vi "App - analyze RUS V6.vi"() -> ()   [LabVIEW 2018] (continued)
"z(inf)"=-0.13064639987627175-0.4414329201397408i, "z (pi/2)"=0.4734329201397408-0.15464639987627177i, "z center"=0.028000000000000025+0.0040000000000000036i, "z(0)"=0.1866463998762718+0.4494329201397408i, "radius"=0.4728415871493524}}, "timestamp(min)"=474.80000000447035, "timestamp"=timestamp(3493756309 s since 1904-01-01), "Magn Field(T)"=0.0}, {"temperature"=120.365, "lorentzian"={"A (VHz)"=0.00010643307998407587, "f (Hz)"=668.3129997886653, "G (Hz)"=0.026481266968947207, "phi(rad)"=2.884384764495416, "Q"=25237.19883086979, "Norm  Ampl"=0.01202799865082056, "bg (V)"=-0.12754197010931823-0.42726620706178137i, "4corners"={"z (-pi/2)"=-0.4512662070617814+0.12754197010931823i, "z(inf)"=-0.12754197010931823-0.42726620706178137i, "z (pi/2)"=0.42726620706178137-0.10354197010931819i, "z center"=-0.01200000000000001+0.01200000000000001i, "z(0)"=0.10354197010931819+0.4512662070617814i, "radius"=0.4542078241545233}}, "timestamp(min)"=476.1166666671634, "timestamp"=timestamp(3493756388 s since 1904-01-01), "Magn Field(T)"=0.0}, {"temperature"=120.108, "lorentzian"={"A (VHz)"=9.976743757357866e-05, "f (Hz)"=668.3140680165973, "G (Hz)"=0.02490702053107623, "phi(rad)"=3.037932161061489, "Q"=26832.35705301438, "Norm  Ampl"=0.011771320920466868, "bg (V)"=-0.020903351691279173-0.4660736150774217i, "4corners"={"z (-pi/2)"=-0.44207361507742166+0.0529033516912792i, "z(inf)"=-0.020903351691279173-0.4660736150774217i, "z (pi/2)"=0.4980736150774217-0.044903351691279195i, "z center"=0.028000000000000025+0.0040000000000000036i, "z(0)"=0.07690335169127922+0.4740736150774217i, "radius"=0.4726105599736393}}, "timestamp(min)"=477.45000000298023, "timestamp"=timestamp(3493756468 s since 1904-01-01), "Magn Field(T)"=0.0}, {"temperature"=119.859, "lorentzian"={"A (VHz)"=0.00011898875098084783, "f (Hz)"=668.3088794677242, "G (Hz)"=0.029414461497605328, "phi(rad)"=3.1937111533621003, "Q"=22720.418645846436, "Norm  Ampl"=0.014251449395847925, "bg (V)"=0.0612402357051023-0.4798469642263822i, "4corners"={"z (-pi/2)"=-0.44784696422638215-0.02124023570510226i, "z(inf)"=0.0612402357051023-0.4798469642263822i, "z (pi/2)"=0.5198469642263822+0.029240235705102268i, "z center"=0.03600000000000003+0.0040000000000000036i, "z(0)"=0.010759764294897767+0.4878469642263822i, "radius"=0.4845048547636392}}, "timestamp(min)"=478.76666666567326, "timestamp"=timestamp(3493756547 s since 1904-01-01), "Magn Field(T)"=0.0}, {"temperature"=119.604, "lorentzian"={"A (VHz)"=0.00010355482355173766, "f (Hz)"=668.3109415026871, "G (Hz)"=0.02529392336725071, "phi(rad)"=3.2924075486690434, "Q"=26421.798303065247, "Norm  Ampl"=0.011934347555654482, "bg (V)"=0.10688904433211106-0.4624709498016203i, "4corners"={"z (-pi/2)"=-0.43047094980162026-0.06688904433211103i, "z(inf)"=0.10688904433211106-0.4624709498016203i, "z (pi/2)"=0.5024709498016203+0.07488904433211103i, "z center"=0.03600000000000003+0.0040000000000000036i, "z(0)"=-0.034889044332111+0.4704709498016203i, "radius"=0.4718266669182082}}, "timestamp(min)"=480.08333333581686, "timestamp"=timestamp(3493756626 s since 1904-01-01), "Magn Field(T)"=0.0}, {"temperature"=119.349, "lorentzian"={"A (VHz)"=8.801887306847703e-05, "f (Hz)"=668.3052156629583, "G (Hz)"=0.021698735780586516, "phi(rad)"=3.2142167974714875, "Q"=30799.26970956895, "Norm  Ampl"=0.010466488120373691, "bg (V)"=0.07099981492336191-0.47708326828925746i, "4corners"={"z (-pi/2)"=-0.4450832682892574-0.03099981492336188i, "z(inf)"=0.07099981492336191-0.47708326828925746i, "z (pi/2)"=0.5170832682892574+0.03899981492336189i, "z center"=0.03600000000000003+0.0040000000000000036i, "z(0)"=0.0010001850766381479+0.48508326828925746i, "radius"=0.48235474297714054}}, "timestamp(min)"=481.41666666418314, "timestamp"=timestamp(3493756706 s since 1904-01-01), "Magn Field(T)"=0.0}, {"temperature"=119.104, "lorentzian"={"A (VHz)"=0.00010821801624048861, "f (Hz)"=668.3064621156966, "G (Hz)"=0.025882538370321603, "phi(rad)"=3.375797533755535, "Q"=25820.74650305609, "Norm  Ampl"=0.012706744245672173, "bg (V)"=0.14993201098301023-0.4735358362984421i, "4corners"={"z (-pi/2)"=-0.44153583629844206-0.1099320109830102i, "z(inf)"=0.14993201098301023-0.4735358362984421i, "z (pi/2)"=0.5135358362984421+0.1179320109830102i, "z center"=0.03600000000000003+0.0040000000000000036i, "z(0)"=-0.07793201098301017+0.4815358362984421i, "radius"=0.49093887407281694}}, "timestamp(min)"=482.73333333432674, "timestamp"=timestamp(3493756785 s since 1904-01-01), "Magn Field(T)"=0.0}, {"temperature"=118.85, "lorentzian"={"A (VHz)"=9.39701073854705e-05, "f (Hz)"=668.2991530946135, "G (Hz)"=0.022918275642981233, "phi(rad)"=3.2389285611028322, "Q"=29160.09753549157, "Norm  Ampl"=0.011143619731764974, "bg (V)"=0.08325322342802156-0.4799313693938589i, "4corners"={"z (-pi/2)"=-0.44793136939385886-0.04325322342802153i, "z(inf)"=0.08325322342802156-0.4799313693938589i, "z (pi/2)"=0.519931369393859+0.051253223428021535i, "z center"=0.03600000000000003+0.0040000000000000036i, "z(0)"=-0.0112532234280215+0.4879313693938589i, "radius"=0.48623290448894346}}, "timestamp(min)"=484.0666666701436, "timestamp"=timestamp(3493756865 s since 1904-01-01), "Magn Field(T)"=0.0}, {"temperature"=118.609, "lorentzian"={"A (VHz)"=0.00010743883910296562, "f (Hz)"=668.296337187602, "G (Hz)"=0.026266437532917148, "phi(rad)"=3.235613845829878, "Q"=25442.975902236147, "Norm  Ampl"=0.012711224583429891, "bg (V)"=0.08143305323019587-0.4777966817581062i, "4corners"={"z (-pi/2)"=-0.44579668175810616-0.041433053230195825i, "z(inf)"=0.08143305323019587-0.4777966817581062i, "z (pi/2)"=0.5177966817581062+0.04943305323019583i, "z center"=0.03600000000000003+0.0040000000000000036i, "z(0)"=-0.009433053230195797+0.4857966817581062i, "radius"=0.4839340914617813}}, "timestamp(min)"=485.3833333328366, "timestamp"=timestamp(3493756944 s since 1904-01-01), "Magn Field(T)"=0.0}, {"temperature"=118.359, "lorentzian"={"A (VHz)"=0.0001070844718829983, "f (Hz)"=668.2941712628873, "G (Hz)"=0.026124370760870142, "phi(rad)"=3.33110736221513, "Q"=25581.25427709356, "Norm  Ampl"=0.012647127694562135, "bg (V)"=0.13519818462181604-0.4714445853921451i, "4corners"={"z (-pi/2)"=-0.4314445853921451-0.08719818462181601i, "z(inf)"=0.13519818462181604-0.4714445853921451i, "z (pi/2)"=0.5194445853921452+0.09519818462181602i, "z center"=0.04400000000000004+0.0040000000000000036i, "z(0)"=-0.04719818462181598+0.47944458539214513i, "radius"=0.48411224179628387}}, "timestamp(min)"=486.70000000298023, "timestamp"=timestamp(3493757023 s since 1904-01-01), "Magn Field(T)"=0.0}, {"temperature"=118.111, "lorentzian"={"A (VHz)"=0.0001130613397389126, "f (Hz)"=668.2879323748828, "G (Hz)"=0.02790011297894843, "phi(rad)"=3.2373022589244065, "Q"=23952.875491189887, "Norm  Ampl"=0.013424939419339223, "bg (V)"=0.08198314261289943-0.47497648031024303i, "4corners"={"z (-pi/2)"=-0.442976480310243-0.04198314261289939i, "z(inf)"=0.08198314261289943-0.47497648031024303i, "z (pi/2)"=0.514976480310243+0.0499831426128994i, "z center"=0.03600000000000003+0.0040000000000000036i, "z(0)"=-0.009983142612899364+0.48297648031024304i, "radius"=0.4811786758522731}}, "timestamp(min)"=488.0333333313465, "timestamp"=timestamp(3493757103 s since 1904-01-01), "Magn Field(T)"=0.0}, {"temperature"=117.87, "lorentzian"={"A (VHz)"=0.00011059651751790313, "f (Hz)"=668.2827006729923, "G (Hz)"=0.027979379247465956, "phi(rad)"=3.139826857303401, "Q"=23884.82942249398, "Norm  Ampl"=0.013390188683237079, "bg (V)"=0.03515493717875207-0.4745727263376128i, "4corners"={"z (-pi/2)"=-0.4425727263376128+0.004845062821247961i, "z(inf)"=0.03515493717875207-0.4745727263376128i, "z (pi/2)"=0.5145727263376129+0.0031549371787520457i, "z center"=0.03600000000000003+0.0040000000000000036i, "z(0)"=0.03684506282124799+0.48257272633761283i, "radius"=0.47857347244220244}}, "timestamp(min)"=489.3500000014901, "timestamp"=timestamp(3493757182 s since 1904-01-01), "Magn Field(T)"=0.0}, {"temperature"=117.621, "lorentzian"={"A (VHz)"=0.00011421298073050124, "f (Hz)"=668.2752935986506, "G (Hz)"=0.02906321623228526, "phi(rad)"=3.0733097507748752, "Q"=22993.85203129336, "Norm  Ampl"=0.01393302684205042, "bg (V)"=0.003290324428110697-0.4742869727474171i, "4corners"={"z (-pi/2)"=-0.4422869727474171+0.03670967557188934i, "z(inf)"=0.003290324428110697-0.4742869727474171i, "z (pi/2)"=0.5142869727474171-0.02870967557188933i, "z center"=0.03600000000000003+0.0040000000000000036i, "z(0)"=0.06870967557188937+0.4822869727474171i, "radius"=0.4794041626601784}}, "timestamp(min)"=490.66666666418314, "timestamp"=timestamp(3493757261 s since 1904-01-01), "Magn Field(T)"=0.0}, {"temperature"=117.382, "lorentzian"={"A (VHz)"=0.00011070346840073388, "f (Hz)"=668.2706731525243, "G (Hz)"=0.028260232808520972, "phi(rad)"=3.0887902740086197, "Q"=23647.033542874018, "Norm  Ampl"=0.013444461231823078, "bg (V)"=0.010891582862682068-0.47107476262981013i, "4corners"={"z (-pi/2)"=-0.4390747626298101+0.029108417137317967i, "z(inf)"=0.010891582862682068-0.47107476262981013i, "z (pi/2)"=0.5110747626298102-0.02110841713731796i, "z center"=0.03600000000000003+0.0040000000000000036i, "z(0)"=0.061108417137317995+0.47907476262981014i, "radius"=0.4757378087759181}}, "timestamp(min)"=492.0, "timestamp"=timestamp(3493757341 s since 1904-01-01), "Magn Field(T)"=0.0}, {"temperature"=117.138, "lorentzian"={"A (VHz)"=0.00010800943974293567, "f (Hz)"=668.265311084802, "G (Hz)"=0.02797683885251187, "phi(rad)"=3.0873037764057782, "Q"=23886.37667778547, "Norm  Ampl"=0.013306749021252626, "bg (V)"=0.010191020561799904-0.4709337312500312i, "4corners"={"z (-pi/2)"=-0.43893373125003116+0.029808979438200132i, "z(inf)"=0.010191020561799904-0.4709337312500312i, "z (pi/2)"=0.5109337312500313-0.021808979438200125i, "z center"=0.03600000000000003+0.0040000000000000036i, "z(0)"=0.06180897943820016+0.4789337312500312i, "radius"=0.4756344736230946}}, "timestamp(min)"=493.3166666701436, "timestamp"=timestamp(3493757420 s since 1904-01-01), "Magn Field(T)"=0.0}, {"temperature"=116.892, "lorentzian"={"A (VHz)"=0.00011678085083385915, "f (Hz)"=668.2583083453824, "G (Hz)"=0.03012977871709603, "phi(rad)"=3.0862999154696142, "Q"=22179.330111249834, "Norm  Ampl"=0.014575891093322855, "bg (V)"=0.00926464512112294-0.47903094309897204i, "4corners"={"z (-pi/2)"=-0.447030943098972+0.030735354878877096i, "z(inf)"=0.00926464512112294-0.47903094309897204i, "z (pi/2)"=0.5190309430989721-0.02273535487887709i, "z center"=0.03600000000000003+0.0040000000000000036i, "z(0)"=0.06273535487887713+0.48703094309897205i, "radius"=0.48377026695693265}}, "timestamp(min)"=494.6499999985099, "timestamp"=timestamp(3493757500 s since 1904-01-01), "Magn Field(T)"=0.0}, {"temperature"=116.657, "lorentzian"={"A (VHz)"=0.00012538810354815837, "f (Hz)"=668.2568309954227, "G (Hz)"=0.032286617496826396, "phi(rad)"=3.2130369520804023, "Q"=20697.64140084073, "Norm  Ampl"=0.015358626788303374, "bg (V)"=0.06195688871592034-0.4704828421346862i, "4corners"={"z (-pi/2)"=-0.4464828421346862-0.02995688871592031i, "z(inf)"=0.06195688871592034-0.4704828421346862i, "z (pi/2)"=0.5024828421346863+0.03795688871592032i, "z center"=0.028000000000000025+0.0040000000000000036i, "z(0)"=-0.005956888715920289+0.4784828421346862i, "radius"=0.4756963714087748}}, "timestamp(min)"=495.9666666686535, "timestamp"=timestamp(3493757579 s since 1904-01-01), "Magn Field(T)"=0.0}, {"temperature"=116.414, "lorentzian"={"A (VHz)"=0.00012730750637721753, "f (Hz)"=668.251544958297, "G (Hz)"=0.03283669747483084, "phi(rad)"=3.262105480773335, "Q"=20350.753770853735, "Norm  Ampl"=0.015732228210800864, "bg (V)"=0.09359864898441411-0.47163017441834365i, "4corners"={"z (-pi/2)"=-0.4396301744183436-0.05359864898441408i, "z(inf)"=0.09359864898441411-0.47163017441834365i, "z (pi/2)"=0.5116301744183437+0.061598648984414084i, "z center"=0.03600000000000003+0.0040000000000000036i, "z(0)"=-0.02159864898441405+0.47963017441834366i, "radius"=0.47910506904232786}}, "timestamp(min)"=497.2833333313465, "timestamp"=timestamp(3493757658 s since 1904-01-01), "Magn Field(T)"=0.0}, {"temperature"=116.182, "lorentzian"={"A (VHz)"=0.00013443649190837575, "f (Hz)"=668.2453085062731, "G (Hz)"=0.035201673002130396, "phi(rad)"=3.27100569161246, "Q"=18983.33946985506, "Norm  Ampl"=0.016690935833129323, "bg (V)"=0.0971902879419883-0.4661868320027308i, "4corners"={"z (-pi/2)"=-0.4341868320027308-0.05719028794198826i, "z(inf)"=0.0971902879419883-0.4661868320027308i, "z (pi/2)"=0.5061868320027308+0.06519028794198826i, "z center"=0.03600000000000003+0.0040000000000000036i, "z(0)"=-0.02519028794198823+0.4741868320027308i, "radius"=0.4741517777328138}}, "timestamp(min)"=498.6166666671634, "timestamp"=timestamp(3493757738 s since 1904-01-01), "Magn Field(T)"=0.0}, {"temperature"=115.94, "lorentzian"={"A (VHz)"=0.0001411771983919197, "f (Hz)"=668.2394743021457, "G (Hz)"=0.0369135267967175, "phi(rad)"=3.2980610919863382, "Q"=18102.83471373882, "Norm  Ampl"=0.017546101039359215, "bg (V)"=0.11007101432524297-0.46552310715567025i, "4corners"={"z (-pi/2)"=-0.4335231071556702-0.07007101432524293i, "z(inf)"=0.11007101432524297-0.46552310715567025i, "z (pi/2)"=0.5055231071556703+0.07807101432524294i, "z center"=0.03600000000000003+0.0040000000000000036i, "z(0)"=-0.0380710143252429+0.47352310715567025i, "radius"=0.4753298468603516}}, "timestamp(min)"=499.933333337307, "timestamp"=timestamp(3493757817 s since 1904-01-01), "Magn Field(T)"=0.0}, {"temperature"=115.7, "lorentzian"={"A (VHz)"=0.0001435934643755886, "f (Hz)"=668.2322266809226, "G (Hz)"=0.03813748540583941, "phi(rad)"=3.3056536907773015, "Q"=17521.664566238192, "Norm  Ampl"=0.01822797887630577, "bg (V)"=0.114062403211538-0.4675364967002526i, "4corners"={"z (-pi/2)"=-0.4355364967002526-0.07406240321153797i, "z(inf)"=0.114062403211538-0.4675364967002526i, "z (pi/2)"=0.5075364967002527+0.08206240321153797i, "z center"=0.03600000000000003+0.0040000000000000036i, "z(0)"=-0.04206240321153794+0.4755364967002526i, "radius"=0.47795439794556555}}, "timestamp(min)"=501.25, "timestamp"=timestamp(3493757896 s since 1904-01-01), "Magn Field(T)"=0.0}, {"temperature"=115.472, "lorentzian"={"A (VHz)"=0.00015015013294900263, "f (Hz)"=668.2226032955875, "G (Hz)"=0.03977315572948954, "phi(rad)"=3.294194856757234, "Q"=16800.84446505557, "Norm  Ampl"=0.019165843957809636, "bg (V)"=0.1092507018179084-0.47227890465981215i, "4corners"={"z (-pi/2)"=-0.4402789046598121-0.06925070181790836i, "z(inf)"=0.1092507018179084-0.47227890465981215i, "z (pi/2)"=0.5122789046598122+0.07725070181790837i, "z center"=0.03600000000000003+0.0040000000000000036i, "z(0)"=-0.037250701817908335+0.48027890465981216i, "radius"=0.4818788855519264}}, "timestamp(min)"=502.58333333581686, "timestamp"=timestamp(3493757976 s since 1904-01-01), "Magn Field(T)"=0.0}, {"temperature"=115.231, "lorentzian"={"A (VHz)"=0.000152798278466846, "f (Hz)"=668.2221912502285, "G (Hz)"=0.040622965881621786, "phi(rad)"=3.3489762299985824, "Q"=16449.369876081317, "Norm  Ampl"=0.019466830319116384, "bg (V)"=0.1346689441843829-0.46493952367230446i, "4corners"={"z (-pi/2)"=-0.4329395236723044-0.09466894418438287i, "z(inf)"=0.1346689441843829-0.46493952367230446i, "z (pi/2)"=0.5049395236723044+0.10266894418438288i, "z center"=0.03600000000000003+0.0040000000000000036i, "z(0)"=-0.06266894418438285+0.47293952367230446i, "radius"=0.4792075097580052}}, "timestamp(min)"=503.8999999985099, "timestamp"=timestamp(3493758055 s since 1904-01-01), "Magn Field(T)"=0.0}, {"temperature"=115.003, "lorentzian"={"A (VHz)"=0.00015016084801885404, "f (Hz)"=668.2178106776172, "G (Hz)"=0.039990622388638174, "phi(rad)"=3.381149177122383, "Q"=16709.36261465803, "Norm  Ampl"=0.019131967464758187, "bg (V)"=0.15751353904588636-0.4607494937776951i, "4corners"={"z (-pi/2)"=-0.42074949377769505-0.10951353904588632i, "z(inf)"=0.15751353904588636-0.4607494937776951i, "z (pi/2)"=0.5087494937776951+0.11751353904588632i, "z center"=0.04400000000000004+0.0040000000000000036i, "z(0)"=-0.06951353904588628+0.4687494937776951i, "radius"=0.47841134551068687}}, "timestamp(min)"=505.23333333432674, "timestamp"=timestamp(3493758135 s since 1904-01-01), "Magn Field(T)"=0.0}, {"temperature"=114.767, "lorentzian"={"A (VHz)"=0.00015757298754621695, "f (Hz)"=668.2137975862624, "G (Hz)"=0.04267438204697135, "phi(rad)"=3.4106089120816963, "Q"=15658.429379264706, "Norm  Ampl"=0.02049382198056047, "bg (V)"=0.16363895936930345-0.458964339411539i, "4corners"={"z (-pi/2)"=-0.426964339411539-0.12363895936930341i, "z(inf)"=0.16363895936930345-0.458964339411539i, "z (pi/2)"=0.49896433941153906+0.13163895936930342i, "z center"=0.03600000000000003+0.0040000000000000036i, "z(0)"=-0.09163895936930339+0.46696433941153903i, "radius"=0.4802371117642215}}, "timestamp(min)"=506.55000000447035, "timestamp"=timestamp(3493758214 s since 1904-01-01), "Magn Field(T)"=0.0}, {"temperature"=114.531, "lorentzian"={"A (VHz)"=0.00015361317354396095, "f (Hz)"=668.2079346540519, "G (Hz)"=0.041298080432760224, "phi(rad)"=3.398310296093033, "Q"=16180.120907604885, "Norm  Ampl"=0.01996843308490766, "bg (V)"=0.16676908728823442-0.463674027337198i, "4corners"={"z (-pi/2)"=-0.42367402733719794-0.11876908728823439i, "z(inf)"=0.16676908728823442-0.463674027337198i, "z (pi/2)"=0.511674027337198+0.12676908728823438i, "z center"=0.04400000000000004+0.0040000000000000036i, "z(0)"=-0.07876908728823435+0.471674027337198i, "radius"=0.48351964245455464}}, "timestamp(min)"=507.8666666671634, "timestamp"=timestamp(3493758293 s since 1904-01-01), "Magn Field(T)"=0.0}, {"temperature"=114.307, "lorentzian"={"A (VHz)"=0.00015578562086982487, "f (Hz)"=668.2000760755379, "G (Hz)"=0.04298628045116837, "phi(rad)"=3.383233224979629, "Q"=15544.496268631594, "Norm  Ampl"=0.02045395031435505, "bg (V)"=0.14186296929284245-0.45800079061954285i, "4corners"={"z (-pi/2)"=-0.43400079061954283-0.10986296929284242i, "z(inf)"=0.14186296929284245-0.45800079061954285i, "z (pi/2)"=0.4900007906195429+0.11786296929284243i, "z center"=0.028000000000000025+0.0040000000000000036i, "z(0)"=-0.0858629692928424+0.46600079061954286i, "radius"=0.475825079529511}}, "timestamp(min)"=509.20000000298023, "timestamp"=timestamp(3493758373 s since 1904-01-01), "Magn Field(T)"=0.0}, {"temperature"=114.072, "lorentzian"={"A (VHz)"=0.00015529053749936577, "f (Hz)"=668.194062828963, "G (Hz)"=0.041694845458546674, "phi(rad)"=3.3543260153288053, "Q"=16025.819390391709, "Norm  Ampl"=0.01973127159447459, "bg (V)"=0.14391430053991824-0.458562662430859i, "4corners"={"z (-pi/2)"=-0.418562662430859-0.0959143005399182i, "z(inf)"=0.14391430053991824-0.458562662430859i, "z (pi/2)"=0.506562662430859+0.10391430053991821i, "z center"=0.04400000000000004+0.0040000000000000036i, "z(0)"=-0.055914300539918166+0.46656266243085903i, "radius"=0.47323047675261354}}, "timestamp(min)"=510.51666666567326, "timestamp"=timestamp(3493758452 s since 1904-01-01), "Magn Field(T)"=0.0}, {"temperature"=113.842, "lorentzian"={"A (VHz)"=0.00016067612699950575, "f (Hz)"=668.1891261636409, "G (Hz)"=0.042796849003211866, "phi(rad)"=3.394809062342997, "Q"=15613.044925655482, "Norm  Ampl"=0.020075211030941627, "bg (V)"=0.15351387700829827-0.45012328964369214i, "4corners"={"z (-pi/2)"=-0.4181232896436921-0.11351387700829825i, "z(inf)"=0.15351387700829827-0.45012328964369214i, "z (pi/2)"=0.4901232896436922+0.12151387700829826i, "z center"=0.03600000000000003+0.0040000000000000036i, "z(0)"=-0.08151387700829822+0.45812328964369214i, "radius"=0.46908152115205964}}, "timestamp(min)"=511.8500000014901, "timestamp"=timestamp(3493758532 s since 1904-01-01), "Magn Field(T)"=0.0}, {"temperature"=113.618, "lorentzian"={"A (VHz)"=0.0001542811582452129, "f (Hz)"=668.1800061469135, "G (Hz)"=0.040982167537354335, "phi(rad)"=3.3443220525752206, "Q"=16304.164623256744, "Norm  Ampl"=0.01923169205406682, "bg (V)"=0.1384844541906579-0.45565943755480826i, "4corners"={"z (-pi/2)"=-0.4156594375548082-0.09048445419065788i, "z(inf)"=0.1384844541906579-0.45565943755480826i, "z (pi/2)"=0.5036594375548082+0.09848445419065789i, "z center"=0.04400000000000004+0.0040000000000000036i, "z(0)"=-0.05048445419065785+0.46365943755480826i, "radius"=0.4692697631607104}}, "timestamp(min)"=513.1666666641831, "timestamp"=timestamp(3493758611 s since 1904-01-01), "Magn Field(T)"=0.0}, {"temperature"=113.387, "lorentzian"={"A (VHz)"=0.0001624912168982803, "f (Hz)"=668.1744243080439, "G (Hz)"=0.044416582325911676, "phi(rad)"=3.3737772248575197, "Q"=15043.355191204013, "Norm  Ampl"=0.020891572072933687, "bg (V)"=0.1442306313832896-0.4537337421361339i, "4corners"={"z (-pi/2)"=-0.42173374213613385-0.10423063138328956i, "z(inf)"=0.1442306313832896-0.4537337421361339i, "z (pi/2)"=0.4937337421361339+0.11223063138328956i, "z center"=0.03600000000000003+0.0040000000000000036i, "z(0)"=-0.07223063138328953+0.4617337421361339i, "radius"=0.47035523624126285}}, "timestamp(min)"=514.4833333343267, "timestamp"=timestamp(3493758690 s since 1904-01-01), "Magn Field(T)"=0.0}, {"temperature"=113.167, "lorentzian"={"A (VHz)"=0.0001556983032149633, "f (Hz)"=668.167621356464, "G (Hz)"=0.042992225411489386, "phi(rad)"=3.348175213684548, "Q"=15541.591879956524, "Norm  Ampl"=0.020129996156841454, "bg (V)"=0.1240404082002707-0.45426853495999503i, "4corners"={"z (-pi/2)"=-0.430268534959995-0.09204040820027067i, "z(inf)"=0.1240404082002707-0.45426853495999503i, "z (pi/2)"=0.48626853495999506+0.10004040820027067i, "z center"=0.028000000000000025+0.0040000000000000036i, "z(0)"=-0.06804040820027064+0.46226853495999504i, "radius"=0.4682241024783483}}, "timestamp(min)"=515.8000000044703, "timestamp"=timestamp(3493758769 s since 1904-01-01), "Magn Field(T)"=0.0}, {"temperature"=112.937, "lorentzian"={"A (VHz)"=0.00016419580746214888, "f (Hz)"=668.1637736220466, "G (Hz)"=0.045224329465811286, "phi(rad)"=3.425485977825887, "Q"=14774.431849280716, "Norm  Ampl"=0.0213288848716954, "bg (V)"=0.1680996752259816-0.44874605720083394i, "4corners"={"z (-pi/2)"=-0.4167460572008339-0.12809967522598156i, "z(inf)"=0.1680996752259816-0.44874605720083394i, "z (pi/2)"=0.48874605720083397+0.13609967522598157i, "z center"=0.03600000000000003+0.0040000000000000036i, "z(0)"=-0.09609967522598153+0.45674605720083394i, "radius"=0.4716241262973202}}, "timestamp(min)"=517.1333333328366, "timestamp"=timestamp(3493758849 s since 1904-01-01), "Magn Field(T)"=0.0}, {"temperature"=112.71, "lorentzian"={"A (VHz)"=0.00017245504712525025, "f (Hz)"=668.1572968562582, "G (Hz)"=0.047433759727580925, "phi(rad)"=3.4412811422325076, "Q"=14086.112943472835, "Norm  Ampl"=0.02252752294707743, "bg (V)"=0.1762088681702268-0.4497577792019217i, "4corners"={"z (-pi/2)"=-0.4177577792019217-0.13620886817022676i, "z(inf)"=0.1762088681702268-0.4497577792019217i, "z (pi/2)"=0.48975777920192176+0.14420886817022677i, "z center"=0.03600000000000003+0.0040000000000000036i, "z(0)"=-0.10420886817022673+0.45775777920192173i, "radius"=0.4749259404368601}}, "timestamp(min)"=518.4500000029802, "timestamp"=timestamp(3493758928 s since 1904-01-01), "Magn Field(T)"=0.0}, {"temperature"=112.492, "lorentzian"={"A (VHz)"=0.00017070211204150683, "f (Hz)"=668.1537550879266, "G (Hz)"=0.04677378805996331, "phi(rad)"=3.473672889865301, "Q"=14284.79032383187, "Norm  Ampl"=0.022093838974345924, "bg (V)"=0.18999264751515837-0.44254858424220067i, "4corners"={"z (-pi/2)"=-0.41054858424220064-0.14999264751515834i, "z(inf)"=0.18999264751515837-0.44254858424220067i, "z (pi/2)"=0.4825485842422007+0.15799264751515835i, "z center"=0.03600000000000003+0.0040000000000000036i, "z(0)"=-0.11799264751515831+0.4505485842422007i, "radius"=0.4723551350175434}}, "timestamp(min)"=519.7666666656733, "timestamp"=timestamp(3493759007 s since 1904-01-01), "Magn Field(T)"=0.0}, {"temperature"=112.266, "lorentzian"={"A (VHz)"=0.00018223977875365084, "f (Hz)"=668.1449838049871, "G (Hz)"=0.049945994320608485, "phi(rad)"=3.5026596091685995, "Q"=13377.348732234572, "Norm  Ampl"=0.02355087112785759, "bg (V)"=0.20257746875969504-0.4451228845478489i, "4corners"={"z (-pi/2)"=-0.40512288454784884-0.170577468759695i, "z(inf)"=0.20257746875969504-0.4451228845478489i, "z (pi/2)"=0.4771228845478489+0.162577468759695i, "z center"=0.03600000000000003-0.0040000000000000036i, "z(0)"=-0.13057746875969498+0.43712288454784887i, "radius"=0.4715267249798276}}, "timestamp(min)"=521.1000000014901, "timestamp"=timestamp(3493759087 s since 1904-01-01), "Magn Field(T)"=0.0}, {"temperature"=112.049, "lorentzian"={"A (VHz)"=0.00017118504286424681, "f (Hz)"=668.135169475204, "G (Hz)"=0.04711813776736462, "phi(rad)"=3.4409139299761327, "Q"=14179.999489240714, "Norm  Ampl"=0.021846821113515342, "bg (V)"=0.18072038464819612-0.4390447280498502i, "4corners"={"z (-pi/2)"=-0.39904472804985014-0.13272038464819608i, "z(inf)"=0.18072038464819612-0.4390447280498502i, "z (pi/2)"=0.4870447280498502+0.14072038464819608i, "z center"=0.04400000000000004+0.0040000000000000036i, "z(0)"=-0.09272038464819604+0.4470447280498502i, "radius"=0.46366053814306474}}, "timestamp(min)"=522.4166666641831, "timestamp"=timestamp(3493759166 s since 1904-01-01), "Magn Field(T)"=0.0}, {"temperature"=111.826, "lorentzian"={"A (VHz)"=0.0001799658759591542, "f (Hz)"=668.1246913482574, "G (Hz)"=0.049217323444046425, "phi(rad)"=3.414889237193867, "Q"=13574.99036102251, "Norm  Ampl"=0.02301194999389016, "bg (V)"=0.17019722104335014-0.44620515508772524i, "4corners"={"z (-pi/2)"=-0.4062051550877252-0.1221972210433501i, "z(inf)"=0.17019722104335014-0.44620515508772524i, "z (pi/2)"=0.4942051550877253+0.1301972210433501i, "z center"=0.04400000000000004+0.0040000000000000036i, "z(0)"=-0.08219722104335006+0.45420515508772524i, "radius"=0.4675579325245449}}, "timestamp(min)"=523.7333333343267, "timestamp"=timestamp(3493759245 s since 1904-01-01), "Magn Field(T)"=0.0}, {"temperature"=111.603, "lorentzian"={"A (VHz)"=0.00017451974083226369, "f (Hz)"=668.121193286822, "G (Hz)"=0.047920841140946836, "phi(rad)"=3.4354084610725897, "Q"=13942.184180818429, "Norm  Ampl"=0.022112608133803717, "bg (V)"=0.16963616531755749-0.4376656445815023i, "4corners"={"z (-pi/2)"=-0.4056656445815023-0.12963616531755745i, "z(inf)"=0.16963616531755749-0.4376656445815023i, "z (pi/2)"=0.47766564458150235+0.13763616531755746i, "z center"=0.03600000000000003+0.0040000000000000036i, "z(0)"=-0.09763616531755742+0.4456656445815023i, "radius"=0.46144031714228817}}, "timestamp(min)"=525.0666666701436, "timestamp"=timestamp(3493759325 s since 1904-01-01), "Magn Field(T)"=0.0}, {"temperature"=111.388, "lorentzian"={"A (VHz)"=0.00018136247232028246, "f (Hz)"=668.1101664128744, "G (Hz)"=0.05012247702670941, "phi(rad)"=3.4571429929100543, "Q"=13329.55205020793, "Norm  Ampl"=0.02324003286140558, "bg (V)"=0.17989361626749142-0.4447717760991525i, "4corners"={"z (-pi/2)"=-0.4047717760991525-0.1478936162674914i, "z(inf)"=0.17989361626749142-0.4447717760991525i, "z (pi/2)"=0.47677177609915256+0.1398936162674914i, "z center"=0.03600000000000003-0.0040000000000000036i, "z(0)"=-0.10789361626749136+0.4367717760991525i, "radius"=0.4636648912826348}}, "timestamp(min)"=526.3833333328366, "timestamp"=timestamp(3493759404 s since 1904-01-01), "Magn Field(T)"=0.0}, {"temperature"=111.168, "lorentzian"={"A (VHz)"=0.00017732924367748604, "f (Hz)"=668.0998885496297, "G (Hz)"=0.04886431968750325, "phi(rad)"=3.424337305450411, "Q"=13672.550704118205, "Norm  Ampl"=0.02270721472310118, "bg (V)"=0.17364755516380617-0.44224762483338026i, "4corners"={"z (-pi/2)"=-0.4022476248333802-0.12564755516380613i, "z(inf)"=0.17364755516380617-0.44224762483338026i, "z (pi/2)"=0.4902476248333803+0.13364755516380614i, "z center"=0.04400000000000004+0.0040000000000000036i, "z(0)"=-0.0856475551638061+0.45024762483338027i, "radius"=0.46469929118666137}}, "timestamp(min)"=527.7166666686535, "timestamp"=timestamp(3493759484 s since 1904-01-01), "Magn Field(T)"=0.0}, {"temperature"=110.956, "lorentzian"={"A (VHz)"=0.0001755500351100679, "f (Hz)"=668.0911411970284, "G (Hz)"=0.04871683645184766, "phi(rad)"=3.448905477042299, "Q"=13713.762835511254, "Norm  Ampl"=0.022606833604015622, "bg (V)"=0.1763730746007246-0.43830500659198746i, "4corners"={"z (-pi/2)"=-0.4063050065919874-0.13637307460072456i, "z(inf)"=0.1763730746007246-0.43830500659198746i, "z (pi/2)"=0.4783050065919875+0.14437307460072457i, "z center"=0.03600000000000003+0.0040000000000000036i, "z(0)"=-0.10437307460072454+0.44630500659198746i, "radius"=0.46404560005370016}}, "timestamp(min)"=529.0333333313465, "timestamp"=timestamp(3493759563 s since 1904-01-01), "Magn Field(T)"=0.0}, {"temperature"=110.737, "lorentzian"={"A (VHz)"=0.00018163078790725488, "f (Hz)"=668.0843412935199, "G (Hz)"=0.05044469627537442, "phi(rad)"=3.4720539578691874, "Q"=13243.896596115665, "Norm  Ampl"=0.023423640340629357, "bg (V)"=0.18666973329833123-0.4352186583969567i, "4corners"={"z (-pi/2)"=-0.4032186583969567-0.1466697332983312i, "z(inf)"=0.18666973329833123-0.4352186583969567i, "z (pi/2)"=0.47521865839695676+0.1546697332983312i, "z center"=0.03600000000000003+0.0040000000000000036i, "z(0)"=-0.11466973329833116+0.44321865839695673i, "radius"=0.46434297498316135}}, "timestamp(min)"=530.3500000014901, "timestamp"=timestamp(3493759642 s since 1904-01-01), "Magn Field(T)"=0.0}, {"temperature"=110.519, "lorentzian"={"A (VHz)"=0.0001812071541479742, "f (Hz)"=668.074848351984, "G (Hz)"=0.04959100517706317, "phi(rad)"=3.468032582893634, "Q"=13471.694029323324, "Norm  Ampl"=0.02311847271252755, "bg (V)"=0.1934922330292432-0.4375636507764309i, "4corners"={"z (-pi/2)"=-0.39756365077643085-0.14549223302924316i, "z(inf)"=0.1934922330292432-0.4375636507764309i, "z (pi/2)"=0.48556365077643093+0.15349223302924317i, "z center"=0.04400000000000004+0.0040000000000000036i, "z(0)"=-0.10549223302924313+0.4455636507764309i, "radius"=0.46618278113104883}}, "timestamp(min)"=531.683333337307, "timestamp"=timestamp(3493759722 s since 1904-01-01), "Magn Field(T)"=0.0}, {"temperature"=110.309, "lorentzian"={"A (VHz)"=0.00018694349041188402, "f (Hz)"=668.0672099835513, "G (Hz)"=0.051848808398743444, "phi(rad)"=3.473847235715632, "Q"=12884.909617319998, "Norm  Ampl"=0.02422816607882838, "bg (V)"=0.1964167197133136-0.43772880401937153i, "4corners"={"z (-pi/2)"=-0.3977288040193715-0.14841671971331355i, "z(inf)"=0.1964167197133136-0.43772880401937153i, "z (pi/2)"=0.4857288040193716+0.15641671971331356i, "z center"=0.04400000000000004+0.0040000000000000036i, "z(0)"=-0.10841671971331351+0.44572880401937154i, "radius"=0.4672849160293441}}, "timestamp(min)"=533.0, "timestamp"=timestamp(3493759801 s since 1904-01-01), "Magn Field(T)"=0.0}, {"temperature"=110.092, "lorentzian"={"A (VHz)"=0.0001795295724214495, "f (Hz)"=668.0546726344026, "G (Hz)"=0.04925847870413864, "phi(rad)"=3.448860296676748, "Q"=13562.22705631941, "Norm  Ampl"=0.022840883312951803, "bg (V)"=0.17624688448219566-0.4379766471865395i, "4corners"={"z (-pi/2)"=-0.4059766471865395-0.13624688448219563i, "z(inf)"=0.17624688448219566-0.4379766471865395i, "z (pi/2)"=0.47797664718653954+0.14424688448219564i, "z center"=0.03600000000000003+0.0040000000000000036i, "z(0)"=-0.1042468844821956+0.4459766471865395i, "radius"=0.4636944524848417}}, "timestamp(min)"=534.3166666701436, "timestamp"=timestamp(3493759880 s since 1904-01-01), "Magn Field(T)"=0.0}, {"temperature"=109.886, "lorentzian"={"A (VHz)"=0.00018425700947939067, "f (Hz)"=668.0432151630731, "G (Hz)"=0.05082571027386269, "phi(rad)"=3.474109311678734, "Q"=13143.804809878216, "Norm  Ampl"=0.02335282091786171, "bg (V)"=0.18598107581107173-0.43030073113085054i, "4corners"={"z (-pi/2)"=-0.3983007311308505-0.1459810758110717i, "z(inf)"=0.18598107581107173-0.43030073113085054i, "z (pi/2)"=0.4703007311308506+0.1539810758110717i, "z center"=0.03600000000000003+0.0040000000000000036i, "z(0)"=-0.11398107581107167+0.43830073113085055i, "radius"=0.45946865852007557}}, "timestamp(min)"=535.6499999985099, "timestamp"=timestamp(3493759960 s since 1904-01-01), "Magn Field(T)"=0.0}, {"temperature"=109.672, "lorentzian"={"A (VHz)"=0.00017864747951855305, "f (Hz)"=668.0317886551247, "G (Hz)"=0.04953081680635286, "phi(rad)"=3.4551378676700635, "Q"=13487.195078306127, "Norm  Ampl"=0.022852422995206817, "bg (V)"=0.17830413376772314-0.4348838990750027i, "4corners"={"z (-pi/2)"=-0.40288389907500266-0.1383041337677231i, "z(inf)"=0.17830413376772314-0.4348838990750027i, "z (pi/2)"=0.4748838990750027+0.1463041337677231i, "z center"=0.03600000000000003+0.0040000000000000036i, "z(0)"=-0.10630413376772307+0.4428838990750027i, "radius"=0.4613778747996692}}, "timestamp(min)"=536.9666666686535, "timestamp"=timestamp(3493760039 s since 1904-01-01), "Magn Field(T)"=0.0}, {"temperature"=109.459, "lorentzian"={"A (VHz)"=0.00018219936447157122, "f (Hz)"=668.0206931728633, "G (Hz)"=0.05023590564749462, "phi(rad)"=3.441928253257153, "Q"=13297.673935857052, "Norm  Ampl"=0.023329381688540478, "bg (V)"=0.17338744962959346-0.43960889542050224i, "4corners"={"z (-pi/2)"=-0.4076088954205022-0.13338744962959342i, "z(inf)"=0.17338744962959346-0.43960889542050224i, "z (pi/2)"=0.4796088954205023+0.14138744962959343i, "z center"=0.03600000000000003+0.0040000000000000036i, "z(0)"=-0.1013874496295934+0.44760889542050225i, "radius"=0.46439655835494964}}, "timestamp(min)"=538.3000000044703, "timestamp"=timestamp(3493760119 s since 1904-01-01), "Magn Field(T)"=0.0}, {"temperature"=109.253, "lorentzian"={"A (VHz)"=0.00018326309436219655, "f (Hz)"=668.0108019958866, "G (Hz)"=0.05071614794503111, "phi(rad)"=3.4752117285047524, "Q"=13171.560322757805, "Norm  Ampl"=0.023314289131758165, "bg (V)"=0.1865360113880276-0.43835512614416294i, "4corners"={"z (-pi/2)"=-0.3983551261441629-0.15453601138802758i, "z(inf)"=0.1865360113880276-0.43835512614416294i, "z (pi/2)"=0.47035512614416297+0.14653601138802758i, "z center"=0.03600000000000003-0.0040000000000000036i, "z(0)"=-0.11453601138802755+0.43035512614416294i, "radius"=0.45970149698726026}}, "timestamp(min)"=539.6166666671634, "timestamp"=timestamp(3493760198 s since 1904-01-01), "Magn Field(T)"=0.0}, {"temperature"=109.04, "lorentzian"={"A (VHz)"=0.00017757199001747914, "f (Hz)"=668.000884305955, "G (Hz)"=0.049458648389355514, "phi(rad)"=3.4510272008382445, "Q"=13506.250293118039, "Norm  Ampl"=0.022916329744467515, "bg (V)"=0.17709732027014569-0.4373371638070479i, "4corners"={"z (-pi/2)"=-0.4053371638070479-0.13709732027014565i, "z(inf)"=0.17709732027014569-0.4373371638070479i, "z (pi/2)"=0.47733716380704794+0.14509732027014566i, "z center"=0.03600000000000003+0.0040000000000000036i, "z(0)"=-0.10509732027014562+0.4453371638070479i, "radius"=0.46334322693297797}}, "timestamp(min)"=540.933333337307, "timestamp"=timestamp(3493760277 s since 1904-01-01), "Magn Field(T)"=0.0}, {"temperature"=108.839, "lorentzian"={"A (VHz)"=0.00018576644631526155, "f (Hz)"=667.994986941211, "G (Hz)"=0.050999984731787976, "phi(rad)"=3.5294667905411465, "Q"=13097.944841635488, "Norm  Ampl"=0.023703220099667917, "bg (V)"=0.21178560895114712-0.42624387552457915i, "4corners"={"z (-pi/2)"=-0.3942438755245791-0.17178560895114708i, "z(inf)"=0.21178560895114712-0.42624387552457915i, "z (pi/2)"=0.4662438755245792+0.1797856089511471i, "z center"=0.03600000000000003+0.0040000000000000036i, "z(0)"=-0.13978560895114706+0.43424387552457916i, "radius"=0.46476916070317653}}, "timestamp(min)"=542.2666666656733, "timestamp"=timestamp(3493760357 s since 1904-01-01), "Magn Field(T)"=0.0}, {"temperature"=108.626, "lorentzian"={"A (VHz)"=0.00018356842807220404, "f (Hz)"=667.9845360403064, "G (Hz)"=0.05033450991062088, "phi(rad)"=3.5013014459529397, "Q"=13270.90573100738, "Norm  Ampl"=0.023343170488430178, "bg (V)"=0.1992445651559475-0.43007977717555057i, "4corners"={"z (-pi/2)"=-0.39807977717555054-0.15924456515594745i, "z(inf)"=0.1992445651559475-0.43007977717555057i, "z (pi/2)"=0.4700797771755506+0.16724456515594746i, "z center"=0.03600000000000003+0.0040000000000000036i, "z(0)"=-0.12724456515594743+0.4380797771755506i, "radius"=0.46376075837195413}}, "timestamp(min)"=543.5833333358169, "timestamp"=timestamp(3493760436 s since 1904-01-01), "Magn Field(T)"=0.0}, {"temperature"=108.42, "lorentzian"={"A (VHz)"=0.00018486571760128093, "f (Hz)"=667.9709114890906, "G (Hz)"=0.050025669695526305, "phi(rad)"=3.524875236743303, "Q"=13352.563105193689, "Norm  Ampl"=0.02302485485986471, "bg (V)"=0.19212229818762863-0.4228652251240987i, "4corners"={"z (-pi/2)"=-0.4068652251240987-0.1681222981876286i, "z(inf)"=0.19212229818762863-0.4228652251240987i, "z (pi/2)"=0.4468652251240987+0.17612229818762862i, "z center"=0.020000000000000018+0.0040000000000000036i, "z(0)"=-0.1521222981876286+0.4308652251240987i, "radius"=0.46026080210424003}}, "timestamp(min)"=544.8999999985099, "timestamp"=timestamp(3493760515 s since 1904-01-01), "Magn Field(T)"=0.0}, {"temperature"=108.218, "lorentzian"={"A (VHz)"=0.00019413444151754428, "f (Hz)"=667.963154410693, "G (Hz)"=0.05282036555617498, "phi(rad)"=3.504436521582954, "Q"=12645.939636678728, "Norm  Ampl"=0.02445731659425036, "bg (V)"=0.19234460873825382-0.43688095954132317i, "4corners"={"z (-pi/2)"=-0.40488095954132314-0.1683446087382538i, "z(inf)"=0.19234460873825382-0.43688095954132317i, "z (pi/2)"=0.4608809595413232+0.1603446087382538i, "z center"=0.028000000000000025-0.0040000000000000036i, "z(0)"=-0.13634460873825377+0.42888095954132316i, "radius"=0.46302815849011425}}, "timestamp(min)"=546.2333333343267, "timestamp"=timestamp(3493760595 s since 1904-01-01), "Magn Field(T)"=0.0}, {"temperature"=108.011, "lorentzian"={"A (VHz)"=0.00018941163976566452, "f (Hz)"=667.9559671880407, "G (Hz)"=0.05074632699436853, "phi(rad)"=3.546421018326184, "Q"=13162.646574641072, "Norm  Ampl"=0.02357785750111181, "bg (V)"=0.21099646855162127-0.4230665647268268i, "4corners"={"z (-pi/2)"=-0.3990665647268268-0.17899646855162124i, "z(inf)"=0.21099646855162127-0.4230665647268268i, "z (pi/2)"=0.4550665647268268+0.18699646855162125i, "z center"=0.028000000000000025+0.0040000000000000036i, "z(0)"=-0.15499646855162122+0.4310665647268268i, "radius"=0.46462195192429023}}, "timestamp(min)"=547.5500000044703, "timestamp"=timestamp(3493760674 s since 1904-01-01), "Magn Field(T)"=0.0}, {"temperature"=107.814, "lorentzian"={"A (VHz)"=0.00019594485148496837, "f (Hz)"=667.9461007473978, "G (Hz)"=0.052096852674853734, "phi(rad)"=3.539980895747111, "Q"=12821.237108432926, "Norm  Ampl"=0.02406600625408001, "bg (V)"=0.1992047884271284-0.4217711298786412i, "4corners"={"z (-pi/2)"=-0.40577112987864117-0.1752047884271284i, "z(inf)"=0.1992047884271284-0.4217711298786412i, "z (pi/2)"=0.4457711298786412+0.1832047884271284i, "z center"=0.020000000000000018+0.0040000000000000036i, "z(0)"=-0.15920478842712837+0.4297711298786412i, "radius"=0.46194741176171406}}, "timestamp(min)"=548.8833333328366, "timestamp"=timestamp(3493760754 s since 1904-01-01), "Magn Field(T)"=0.0}, {"temperature"=107.607, "lorentzian"={"A (VHz)"=0.00019261254803453333, "f (Hz)"=667.9364915226823, "G (Hz)"=0.051233485498933584, "phi(rad)"=3.552653666607666, "Q"=13037.108153349927, "Norm  Ampl"=0.023499620420623275, "bg (V)"=0.203279147977592-0.4164679847558972i, "4corners"={"z (-pi/2)"=-0.4004679847558972-0.17927914797759198i, "z(inf)"=0.203279147977592-0.4164679847558972i, "z (pi/2)"=0.4404679847558972+0.187279147977592i, "z center"=0.020000000000000018+0.0040000000000000036i, "z(0)"=-0.16327914797759197+0.4244679847558972i, "radius"=0.45867698033373927}}, "timestamp(min)"=550.2000000029802, "timestamp"=timestamp(3493760833 s since 1904-01-01), "Magn Field(T)"=0.0}, {"temperature"=107.403, "lorentzian"={"A (VHz)"=0.00019585615585340505, "f (Hz)"=667.9270848813279, "G (Hz)"=0.05140542836663986, "phi(rad)"=3.529879382023881, "Q"=12993.318139817055, "Norm  Ampl"=0.023595886932381915, "bg (V)"=0.19378474353100264-0.42084593191813147i, "4corners"={"z (-pi/2)"=-0.40484593191813145-0.16978474353100262i, "z(inf)"=0.19378474353100264-0.42084593191813147i, "z (pi/2)"=0.4448459319181315+0.17778474353100263i, "z center"=0.020000000000000018+0.0040000000000000036i, "z(0)"=-0.1537847435310026+0.4288459319181315i, "radius"=0.45901547136400744}}, "timestamp(min)"=551.5166666656733, 
